vi "temperature_liquid_inlet.vi"(2 "Offset [C]":dbl, 4 "Temp. Voltage\n[V]":dynamicdata(graph)) -> (0 "Offset Temp. [C]":dbl, 1 "Temp. [C]":dbl)   [LabVIEW 2017]
uses:
  <vilib>/express/express shared/transition.llb/Dynamic To Waveform Array.vi
  <vilib>/express/express arith-compare/Formula/Block/exnFormulaBlock how many pts in the wave.vi
  <vilib>/express/express shared/ex_Modify Signal Name.vi
  <vilib>/express/express shared/transition.llb/Waveform Array To Dynamic.vi
  <vilib>/express/express arith-compare/Formula/XNode/ExpressFormulaBlockNode.xnode
panel:
  in  "Temp. Voltage\n[V]":dbl
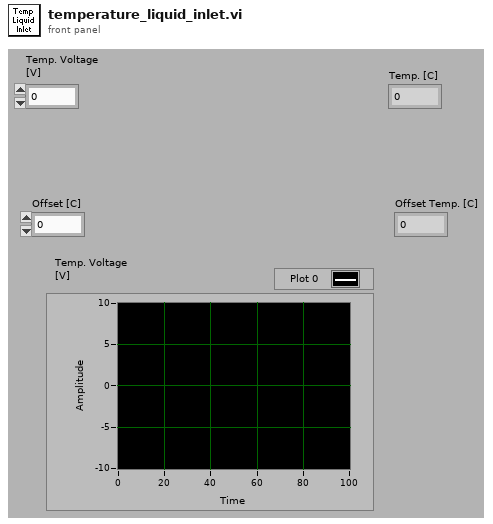
[diagram p1: front panel]
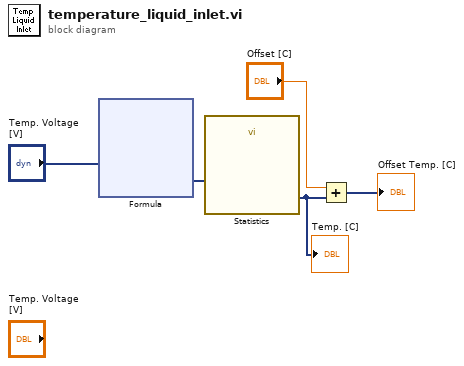
[diagram p0: block diagram]
diagram:
  n1 = xnode "Formula"("V"="Temp. Voltage\n[V]") -> ("Result"=w5:dynamicdata)  [unwired: 1 in, 1 out]
  n2 = call "Statistics"("Signals"=w5) -> ("Arithmetic Mean"=w1:dynamicdata)  [unwired: 25 in, 1 out]
  "Temp. [C]" <- w1
  n3 = Add(x="Offset [C]", y=w1) -> (x+y=→"Offset Temp. [C]":dynamicdata)
